vi "GetTimestamp.vi"(9 "Error in":errorcluster) -> (1 "Timestamp":timestamp)   [LabVIEW 2017, in "GPError.lvlib"]
doc: "Returns <B>Timestamp</B> from <B>Error in</B> if any is set. For appended errors the timestamp from the primary error/warning is returned only.\n\nThis VI is inlined.\n\nSteen Schmidt\nGPower\n17/7 2013"
uses:
  GPError.lvlib
  <vilib>/Utility/miscctls.llb/LVDateTimeRec.ctl
panel:
  # "Copyright © 2014\nGPower\nSee enclosed license file for terms and conditions"
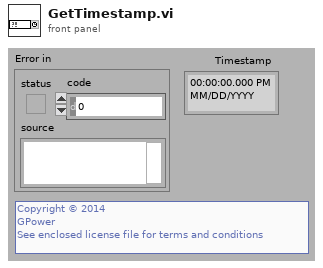
[diagram p1: front panel]
types:
  T1 = typedef "LVDateTimeRec.ctl" = cluster{"fractional second":dbl, "second":i32, "minute":i32, "hour":i32, "day of month":i32, "month":i32, "year":i32, "day of week":i32, "day of year":i32, "DST":i32}
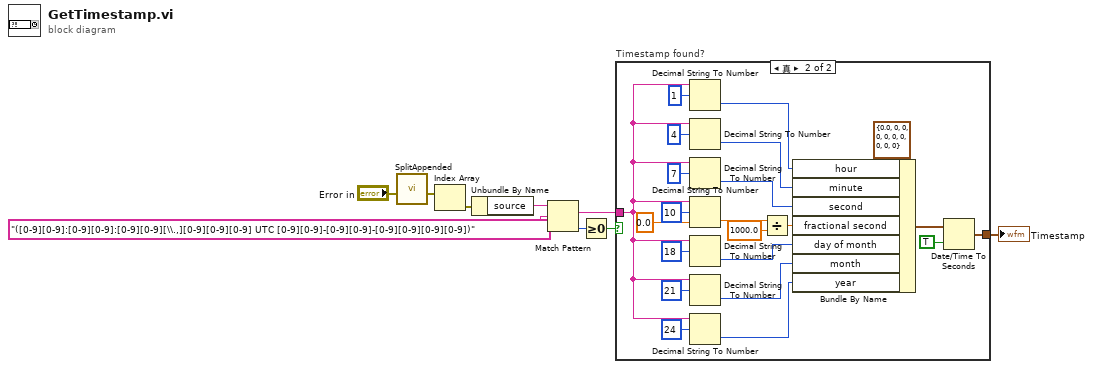
[diagram p0: block diagram]
diagram:
  n1 = call "SplitAppended.vi"("Appended errors in"="Error in") -> ("Errors out"=w8:errorcluster[])  [unwired: 10 in]
  n2 = Index Array(array=w8) -> (element=w5:errorcluster)  [unwired: 1 in]
  n3 = Unbundle By Name(w5) -> ("source"=w7:string)
  n4 = Match Pattern(string=w7, regular expression="([0-9][0-9]:[0-9][0-9]:[0-9][0-9][\\.,][0-9][0-9][0-9] UTC [0-9][0-9]-[0-9][0-9]-[0-9][0-9][0-9][0-9])" ("time format string (%c)")) -> (match substring=w2:string, offset past match=w6:i32)  [unwired: 1 in, 2 out]
  n5 = Greater Or Equal To 0?(x=w6) -> (x >= 0?=w3:bool)
  n6 = case "Timestamp found?" shown="真" w3 {
    tunnel: w2 -> [_ w30]
    tunnel: [_ w10] -> w1
    frame False {
    }
    frame True {
      n7 = Decimal String To Number(string=w30, offset=1 ("offset (0)")) -> (number=w22:i32)  [unwired: 1 in, 1 out]
      n8 = Decimal String To Number(string=w30, offset=4) -> (number=w21:i32)  [unwired: 1 in, 1 out]
      n9 = Decimal String To Number(string=w30, offset=7) -> (number=w20:i32)  [unwired: 1 in, 1 out]
      n10 = Decimal String To Number(string=w30, offset=10, default (0L)=0.0 ("default (0 I32)")) -> (number=w25:dbl)  [unwired: 1 out]
      n11 = Decimal String To Number(string=w30, offset=18) -> (number=w13:i32)  [unwired: 1 in, 1 out]
      n12 = Decimal String To Number(string=w30, offset=21) -> (number=w14:i32)  [unwired: 1 in, 1 out]
      n13 = Decimal String To Number(string=w30, offset=24) -> (number=w15:i32)  [unwired: 1 in, 1 out]
      n14 = Divide(x=w25, y=1000.0) -> (x/y=w23:dbl)
      n15 = Bundle By Name(cluster=T1 {"fractional second"=0.0, "second"=0, "minute"=0, "hour"=0, "day of month"=0, "month"=0, "year"=0, "day of week"=0, "day of year"=0, "DST"=0} ("date time rec"), "hour"=w22, "minute"=w21, "second"=w20, "fractional second"=w23, "day of month"=w13, "month"=w14, "year"=w15) -> (w12:T1)
      n16 = Date/Time To Seconds(1:TRUE ("is UTC (F)"), 2:w12) -> (0:w10:timestamp)
    }
  }
  "Timestamp" <- w1
